vi "Close File.vi"(8 "error in":errorcluster, 11 "File Obs in":refnum<class "File Observer.lvclass">) -> (0 "error out":errorcluster, 3 "File Obs out":refnum<class "File Observer.lvclass">)   [LabVIEW 2015, in "File Observer.lvclass"]
uses:
  File Observer.lvclass
  File Observer.lvclass/File Observer.ctl
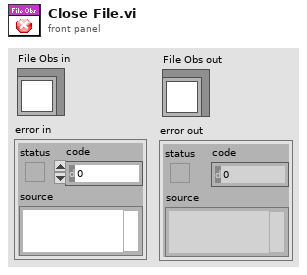
[diagram p1: front panel]
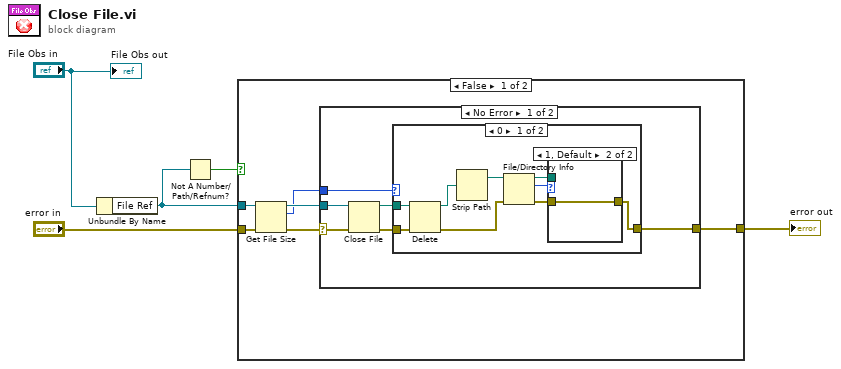
[diagram p0: block diagram]
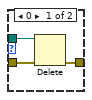
[diagram p2: hidden frame]
diagram:
  n1 = Unbundle By Name("File Obs in") -> ("File Ref"=w2:refnum<file>)
  n2 = Not A Number/Path/Refnum?(number/path/refnum=w2) -> (NaN/Path/Refnum?=w1:bool)
  n3 = case shown="False" w1 {
    tunnel: "error in" -> [w11 w33]
    tunnel: [w10 w33] -> w4
    tunnel: w2 -> [w6 _]
    frame False {
      n4 = Get File Size(file=w6, error in=w11) -> (refnum out=w9:refnum<file>, size (in bytes)=w8:i64, 0:w7:errorcluster)
      n5 = case shown="No Error" w7 {
        selector: w7 -> [w12 w32]
        tunnel: [w17 w32] -> w10
        tunnel: w9 -> [w16 _]
        tunnel: w8 -> [w15 _]
        frame No Error {
          n6 = Close File(refnum=w16, error in=w12) -> (path=w13:path, error out=w14:errorcluster)
          n7 = case shown="0" w15 {
            tunnel: w14 -> [w26 w31]
            tunnel: w13 -> [w25 _]
            tunnel: [w18 w31] -> w17
            frame 0 {
              n8 = Delete(path (use dialog)=w25, error in=w26) -> (deleted path=w24:path, error out=w19:errorcluster)  [unwired: 3 in, 1 out]
              n9 = Strip Path(path=w24) -> (stripped path=w23:path)  [unwired: 1 out]
              n10 = File/Directory Info(path=w23, error in=w19) -> (path out=w20:path, size=w22:i64, error out=w21:errorcluster)  [unwired: 4 out]
              n11 = case shown="1, Default" w22 {
                tunnel: w21 -> [w29 w30]
                tunnel: w20 -> [w28 _]
                tunnel: [w27 w30] -> w18
                frame 0 {
                  n12 = Delete(path (use dialog)=w28, error in=w29) -> (error out=w27:errorcluster)  [unwired: 3 in, 2 out]
                }
                frame 1, Default {
                }
              }
            }
            frame 1, Default {
            }
          }
        }
        frame Error {
        }
      }
    }
    frame True {
    }
  }
  "error out" <- w4
  "File Obs out" <- "File Obs in"
